vi "Tank_Demo.vi"   [LabVIEW 2012, in "Serenity_mk2.lvrbt"]
uses:
  Serenity_mk2.lvrbt
  <vilib>/NXT/Hardware/Plugins/Tetrix 180 deg Servo/Tetrix180ServoAddress.ctl
  <vilib>/NXT/Hardware/Plugins/Tetrix DC Motor/TetrixDCMotorAddress.ctl
  <vilib>/NXT/NXTIO Xnodes/NXTIONodeSubVIs/TETRIX IO Move Servos.vi
  <vilib>/FTC/FTC Calculate Drive Power - Tank.vi
  <vilib>/NXT/NXTIO Xnodes/NXTIONodeSubVIs/TETRIX IO Move DC Motors.vi
  <vilib>/NXT/NXTIO Xnodes/NXTIONodeSubVIs/TETRIX IO Check Battery.vi
  <vilib>/NXT/NXTIO Xnodes/NXTIONodeSubVIs/TETRIX IO Stop DC Motors.vi
  <vilib>/NXT/NXTIO Xnodes/AddressXNode/NXTIOAddress.xnode
  MecanumDrive/Mecanum Drive.lvrbt
  <vilib>/NXT/Subs/LVHSConnector.ctl
  <vilib>/NXT/NXTIO Xnodes/NXTIOXNode/NXTIO.xnode
  <vilib>/NXT/LegoClasses/BrickReference/BrickReference.lvclass
panel:
  # "This VI was generated based on your configuration in the Remote Control Editor. You may modify the code as needed for your robot. To test this program for an FTC match, return to the Remote Control Editor, select the \"Run Program\" tab, and choose \"Teleop\"."
types:
  T1 = typedef "Tetrix180ServoAddress.ctl" = i32
  T2 = typedef "LVHSConnector.ctl" = refnum<class "BrickReference.lvclass">
  T3 = typedef "TetrixDCMotorAddress.ctl" = i32
  T4 = cluster{"TetrixDCMotor":T3, "TetrixDCMotor 2":T3}
  T5 = typedef "FTC ControllerState.ctl" = cluster{"Left X":i8, "Left Y":i8, "Right X":i8, "Right Y":i8, "Button Encoding 9-12":u8, "Button Encoding 1-8":u8, "POV":T6}
  T6 = typedef "FTC POVState.ctl" = i8
  T7 = typedef "FTC ButtonEventType.ctl" = enum16{"Pressed", "Released"}
  T8 = cluster{"Button ID":enum16{"None", "Button 1", "Button 2", "Button 3", "Button 4", "Button 5", "Button 6", "Button 7", "Button 8", "Button 9", "Button 10", "Button 11", "Button 12", "POV Up", "POV Up Right", "POV Right", "POV Down Right", "POV Down", "POV Down Left", "POV Left", "POV Up Left"}, "Event Type":T7}[]
  T9 = typedef "FTC ButtonState.ctl" = cluster{"Button 1":bool, "Button 2":bool, "Button 3":bool, "Button 4":bool, "Button 5":bool, "Button 6":bool, "Button 7":bool, "Button 8":bool, "Button 9":bool, "Button 10":bool, "Button 11":bool, "Button 12":bool, "POV":T6}
  T10 = enum16{"None", "Button 1", "Button 2", "Button 3", "Button 4", "Button 5", "Button 6", "Button 7", "Button 8", "Button 9", "Button 10", "Button 11", "Button 12", "POV Up", "POV Up Right", "POV Right", "POV Down Right", "POV Down", "POV Down Left", "POV Left", "POV Up Left"}
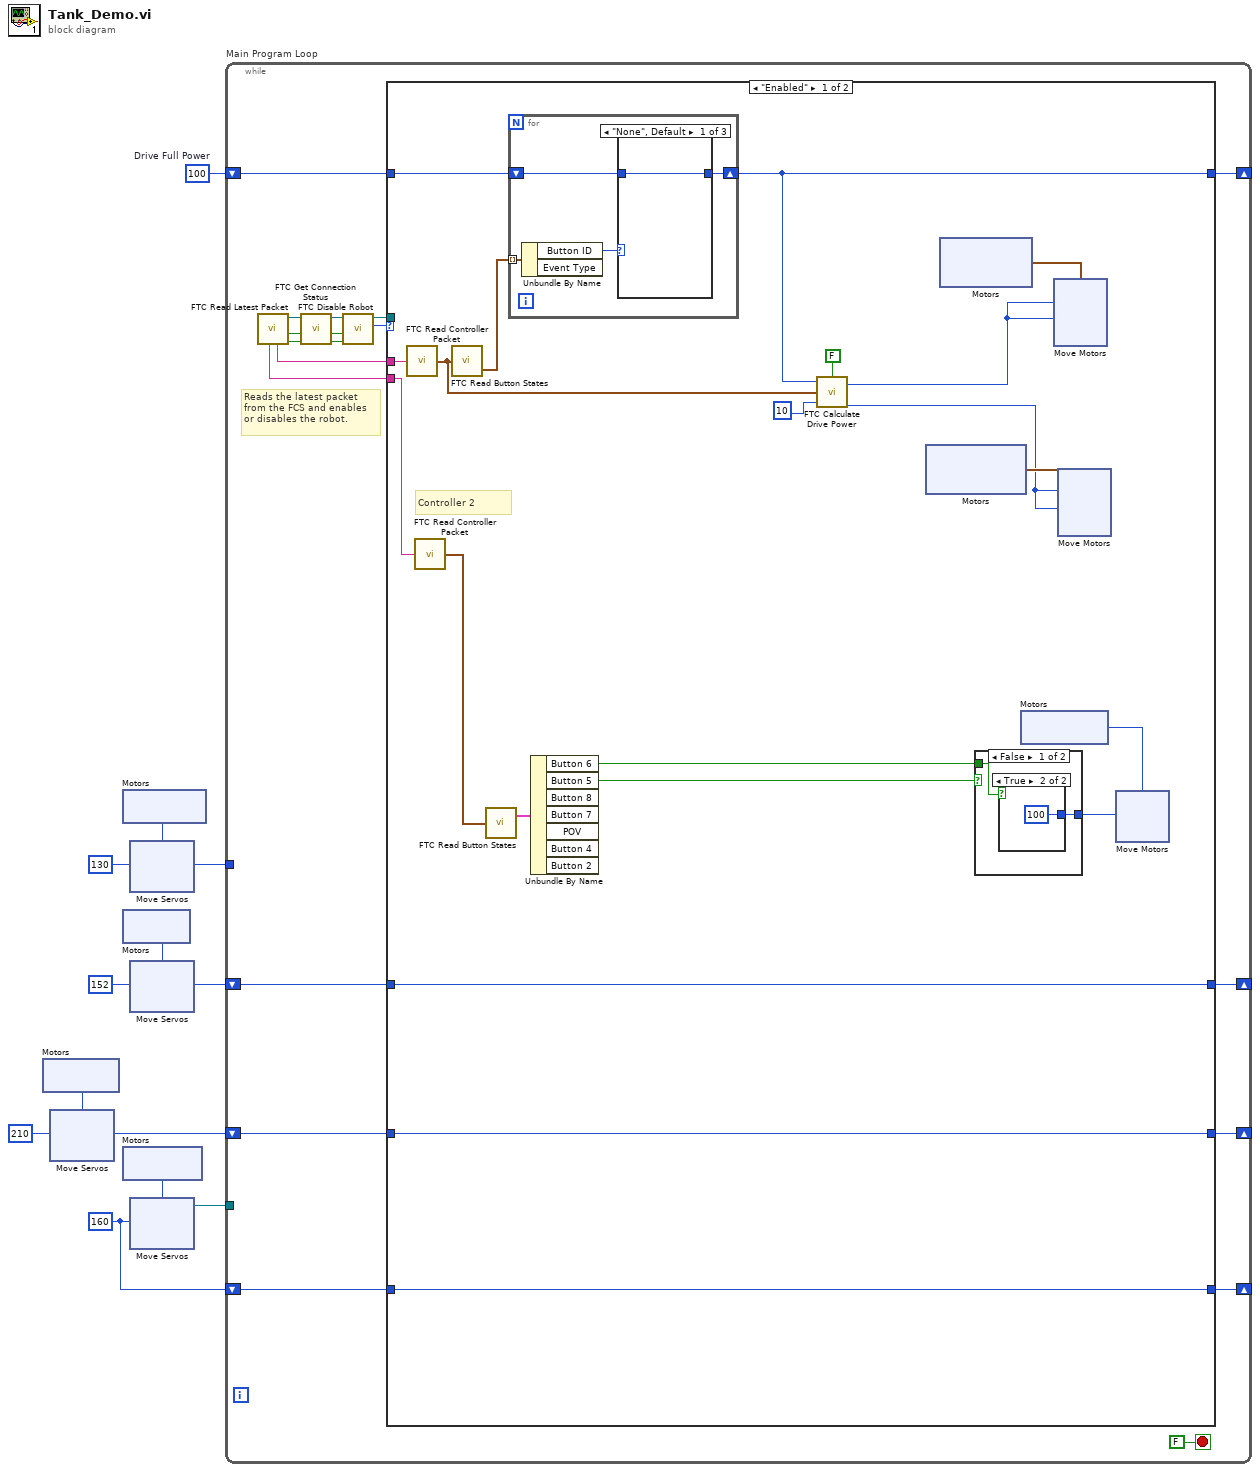
[diagram p0: block diagram]
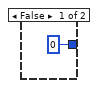
[diagram p2: hidden frame]
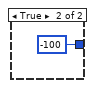
[diagram p3: hidden frame]
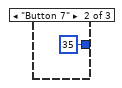
[diagram p4: hidden frame]
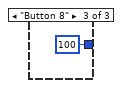
[diagram p5: hidden frame]
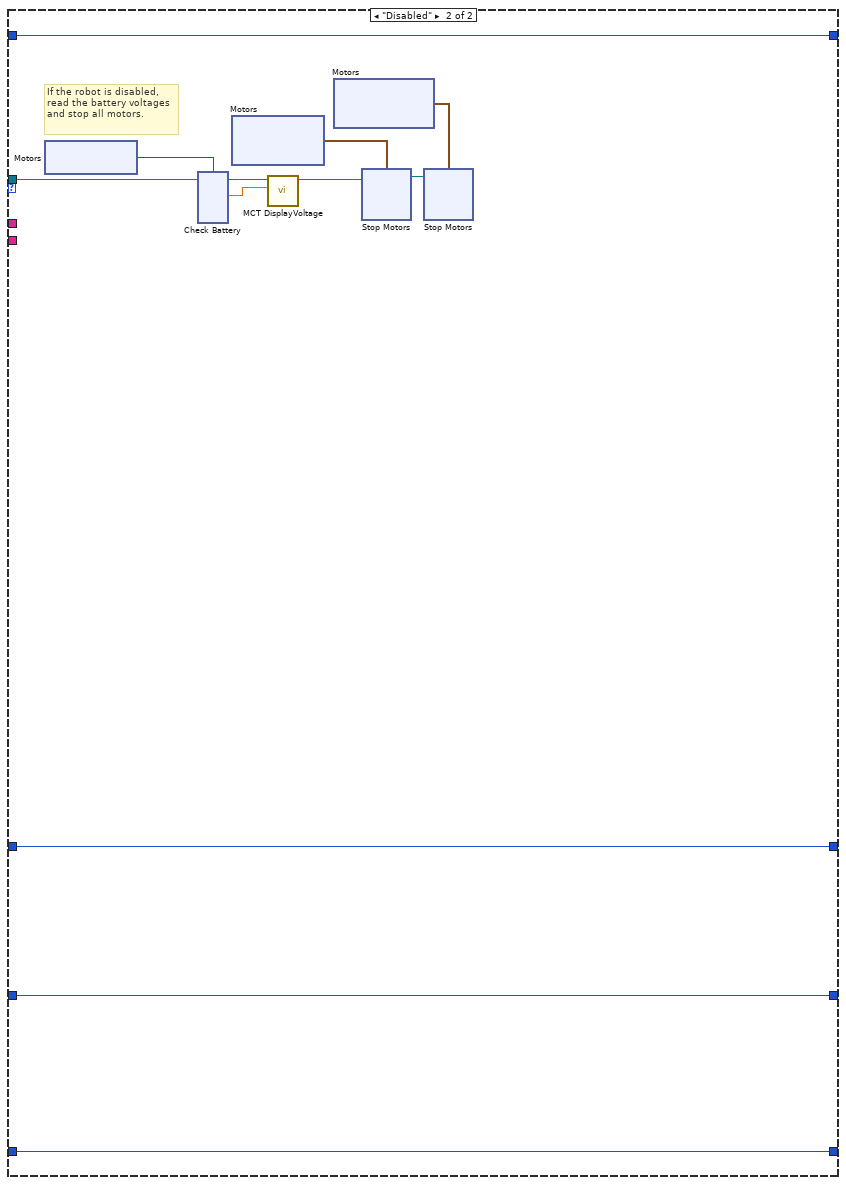
[diagram p6: hidden frame]
diagram:
  w3 = u8 130 ("Position 1")
  w2 = u8 152 ("Position 1")
  w1 = u8 210 ("Position 1")
  w7 = u8 160 ("Position 1")
  w10 = i8 100  # Drive Full Power
  n1 = xnode "Motors"() -> ("Motor"=w6:T1)
  n2 = xnode "Move Servos"("Position 1"=w1, "Motors"=w6) -> ()  [unwired: 1 in, 1 out]
  n3 = xnode "Motors"() -> ("Motor"=w4:T1)
  n4 = xnode "Motors"() -> ("Motor"=w5:T1)
  n5 = xnode "Motors"() -> ("Motor"=w8:T1)
  n6 = xnode "Move Servos"("Position 1"=w3, "Motors"=w4) -> ()  [unwired: 1 in, 1 out]
  n7 = xnode "Move Servos"("Position 1"=w2, "Motors"=w5) -> ()  [unwired: 1 in, 1 out]
  n8 = xnode "Move Servos"("Position 1"=w7, "Motors"=w8) -> ("NXT/EV3"=w9:T2)  [unwired: 1 in]
  n9 = while "Main Program Loop" {
    shift-right: [w17] -> _
    shift-left: w10 -> [w18]
    tunnel: w9 -> [_]
    shift-right: [w16] -> _
    shift-left: w7 -> [w15]
    tunnel: w3 -> [_]
    shift-right: [w11] -> _
    shift-left: w1 -> [w14]
    shift-right: [w12] -> _
    shift-left: w2 -> [w13]
    stop <- FALSE stop-if-true
    # "Reads the latest packet\nfrom the FCS and enables\nor disables the robot."
    n10 = call <vilib>:"FTC Read Latest Packet.vi"() -> ("Packet Received?"=w26:bool, "Stopped?"=w23:bool, "NXT"=w25:T2, "Controller 1"=w28:string, "Controller 2"=w27:string)  [unwired: 6 in, 1 out]
    n11 = call <vilib>:"FTC Get Connection Status.vi"("Packet Received?"=w26, "Stopped?"=w23, "NXT"=w25) -> ("Online?"=w20:bool, "Stopped?"=w21:bool, "NXT"=w22:T2)  [unwired: 5 in]
    n12 = call <vilib>:"FTC Disable Robot.vi"("Online?"=w20, "Stopped?"=w21, "NXT"=w22) -> ("Enabled?"=w24:enum16{"Disabled", "Enabled"}, "NXT"=w19:T2)  [unwired: 3 in]
    n13 = case "disableCase" shown="\"Enabled\"" w24 {
      tunnel: w28 -> [w50 _]
      tunnel: w27 -> [w49 _]
      tunnel: w19 -> [_ w100]
      tunnel: w18 -> [w47 w92]
      tunnel: [w32 w92] -> w17
      tunnel: [w34 w91] -> w16
      tunnel: w15 -> [w34 w91]
      tunnel: w14 -> [w33 w89]
      tunnel: [w35 w90] -> w12
      tunnel: w13 -> [w35 w90]
      tunnel: [w33 w89] -> w11
      frame "Enabled" {
        # "Controller 2"
        n14 = call <vilib>:"FTC Read Controller Packet.vi"("Packet"=w50) -> ("Controller State"=w42:T5)  [unwired: 4 in]
        n15 = call <vilib>:"FTC Read Controller Packet.vi"("Packet"=w49) -> ("Controller State"=w46:T5)  [unwired: 4 in]
        n16 = call <vilib>:"FTC Read Button States.vi"("Controller State"=w42) -> ("Button Events"=w48:T8)  [unwired: 2 in, 1 out]
        n17 = call <vilib>:"FTC Read Button States.vi"("Controller State"=w46) -> ("Button States"=w43:T9)  [unwired: 2 in, 1 out]
        n18 = for {
          tunnel: w48 -> [w85] mode=indexing
          shift-right: [w82] -> w32
          shift-left: w47 -> [w83]
          n19 = Unbundle By Name(w85) -> ("Button ID"=w84:T10)  [unwired: 1 out]
          n20 = case shown="\"None\", Default" w84 {
            tunnel: w83 -> [w86 _ _]
            tunnel: [w86 i8 35 i8 100] -> w82
            frame "None", Default {
            }
            frame "Button 7" {
            }
            frame "Button 8" {
            }
          }
        }
        n21 = Unbundle By Name(w43) -> ("Button 6"=w30:bool, "Button 5"=w31:bool)  [unwired: 5 out]
        n22 = call-poly <vilib>:"FTC Calculate Drive Power.vi"("Reverse"=FALSE, "Deadband (10)"=i8 10, "Controller State"=w42, "Power Level (50)"=w32) -> ("Right Motor Power"=w36:i8, "Left Motor Power"=w37:i8)
        n23 = xnode ("Motors")() -> ("Motor"=w39:cluster{"TetrixDCMotor":T3, "TetrixDCMotor":T3})
        n24 = xnode ("Motors")() -> ("Motor"=w38:cluster{"TetrixDCMotor":T3, "TetrixDCMotor":T3})
        n25 = case shown="False" w31 {
          tunnel: w30 -> [w78 _]
          tunnel: [w77 i8 -100] -> w44
          frame False {
            n26 = case shown="True" w78 {
              tunnel: [i8 0 i8 100] -> w77
              frame False {
              }
              frame True {
              }
            }
          }
          frame True {
          }
        }
        n27 = xnode "Motors"() -> ("Motor"=w45:T3)
        n28 = xnode ("Move Motors")("Power/Speed 2"=w37, "Power/Speed 1"=w37, "Motors"=w38) -> ()  [unwired: 1 in, 1 out]
        n29 = xnode ("Move Motors")("Power/Speed 2"=w36, "Power/Speed 1"=w36, "Motors"=w39) -> ()  [unwired: 1 in, 1 out]
        n30 = xnode "Move Motors"("Power/Speed 1"=w44, "Motors"=w45) -> ()  [unwired: 1 in, 1 out]
      }
      frame "Disabled" {
        # "If the robot is disabled, read the battery voltages and stop all motors."
        n31 = xnode ("Motors")() -> ("Motor"=w99:T3)
        n32 = xnode ("Check Battery")("Motors"=w99, "NXT/EV3"=w100) -> ("Voltage 1"=w98:sgl, "NXT/EV3"=w97:T2)
        n33 = xnode "Motors"() -> ("Motor"=w96:cluster{"TetrixDCMotor":T3, "TetrixDCMotor":T3})
        n34 = call <vilib>:"MCT DisplayVoltage.vi"("Motor Voltage"=w98, "NXT"=w97) -> ("NXT"=w95:T2)  [unwired: 9 in]
        n35 = xnode "Motors"() -> ("Motor"=w94:cluster{"TetrixDCMotor":T3, "TetrixDCMotor":T3})
        n36 = xnode "Stop Motors"("Motors"=w96, "NXT/EV3"=w95) -> ("NXT/EV3"=w93:T2)
        n37 = xnode "Stop Motors"("Motors"=w94, "NXT/EV3"=w93) -> ()  [unwired: 1 out]
      }
    }
  }
